vi "CCE RRMA P01 SubVI01.vi"(0 "imagen":u8, 1 "umbral superior":u8, 2 "umbral inferior":u8=50) -> (7 "umbralizado":u8)   [LabVIEW 2020]
doc: "Ceballos Conde Emanuel Rodríguez Ramírez Miguel Ángel 4MV6 Sistemas de visión artificial 2022/1\nEste vi contiene la operacion de binarizacion para el elemento de entrada, obteninendo a la salida 1 si el valor si encuentra dentro del rango dado por el umbral superior e inferior y 0 cuando se encuentra fuera de este rango"
panel:
  # "Ceballos Conde Emanuel\nRodríguez Ramírez Miguel Ángel\n4MV6\nSistemas de visión artificial\n2022/1"
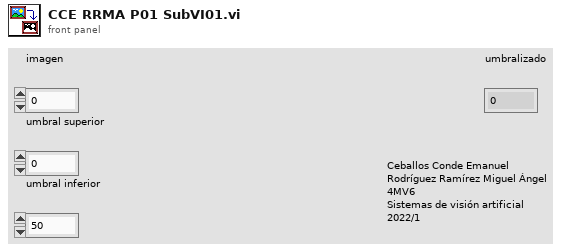
[diagram p1: front panel]
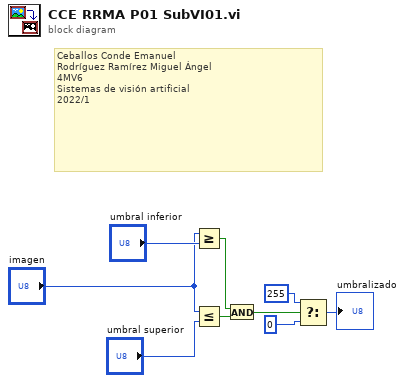
[diagram p0: block diagram]
diagram:
  # "Ceballos Conde Emanuel\nRodríguez Ramírez Miguel Ángel\n4MV6\nSistemas de visión artificial\n2022/1"
  n1 = Greater Or Equal?(x="imagen", y="umbral inferior") -> (x >= y?=w6:bool)
  n2 = Less Or Equal?(x="imagen", y="umbral superior") -> (x <= y?=w4:bool)
  n3 = And(x=w6, y=w4) -> (x .and. y?=w5:bool)
  n4 = Select(t=u8 255, s=w5, f=u8 0) -> (s? t:f=→"umbralizado":u8)
